vi "reset.vi"(8 "error in (no error)":errorcluster, 11 "DataCollectionDL110128Streaming in":refnum<class "DataCollectionDL110128Streaming.lvclass">) -> (0 "error out":errorcluster, 3 "DataCollectionDL110128Streaming out":refnum<class "DataCollectionDL110128Streaming.lvclass">)   [LabVIEW 2010, in "DataCollectionDL110128Streaming.lvclass"]
uses:
  DataCollectionDL110128Streaming.lvclass
  DataCollectionDL091104Scaffold/DataCollectionDL091104Scaffold/DataCollectionDL091104Scaffold.lvclass
  DataCollectionDL110128Streaming.lvclass/DataCollectionDL110128Streaming.ctl
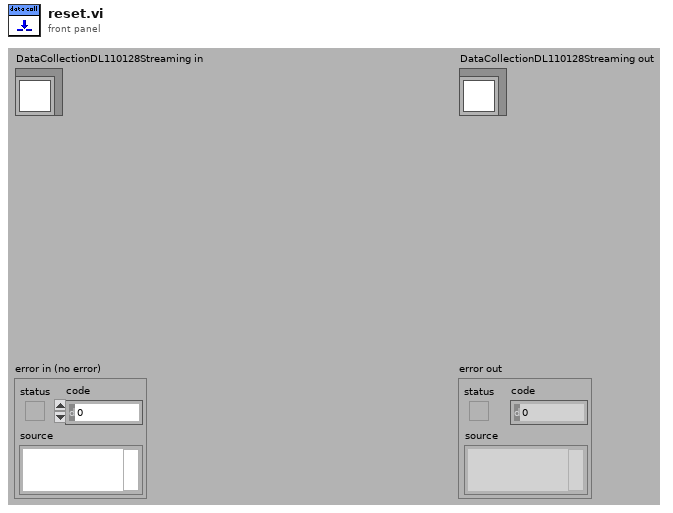
[diagram p1: front panel]
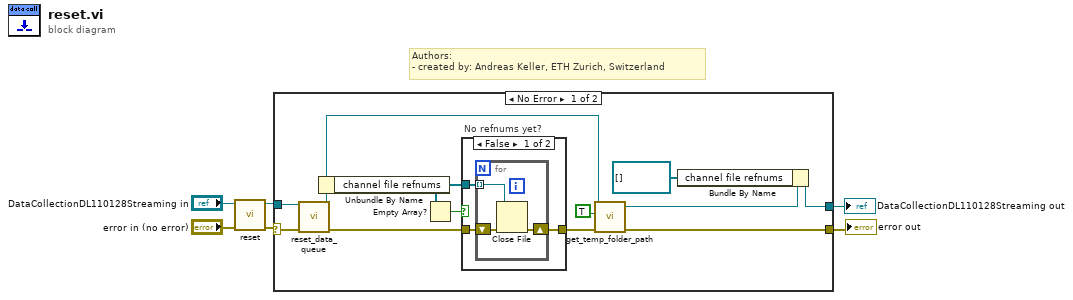
[diagram p0: block diagram]
diagram:
  # "Authors: \n- created by: Andreas Keller, ETH Zurich, Switzerland"
  n1 = call-parent "reset.vi"("error in (no error)"="error in (no error)", "DataCollectionDL091104Scaffold in"="DataCollectionDL110128Streaming in") -> ("error out"=w4:errorcluster, "DataCollectionDL091104Scaffold out"=w3:refnum<class "DataCollectionDL110128Streaming.lvclass">)  [unwired: 8 in]
  n2 = case shown="No Error" w4 {
    selector: w4 -> [w17 w27]
    tunnel: [w11 w27] -> w1
    tunnel: [w8 w26] -> w2
    tunnel: w3 -> [w18 w26]
    frame No Error {
      n3 = call-dynamic "reset_data_queue.vi"("error in (no error)"=w17, "GenericToplevelComponent in"=w18) -> ("error out"=w16:errorcluster, "GenericToplevelComponent out"=w10:refnum<class "DataCollectionDL110128Streaming.lvclass">)  [unwired: 8 in]
      n4 = Unbundle By Name(w10) -> ("channel file refnums"=w12:refnum<file>[])
      n5 = Empty Array?(array=w12) -> (empty?=w13:bool)
      n6 = case "No refnums yet?" shown="False" w13 {
        tunnel: w16 -> [w21 w25]
        tunnel: [w19 w25] -> w14
        tunnel: w12 -> [w20 _]
        frame False {
          n7 = for {
            tunnel: w20 -> [w23] mode=indexing
            shift-right: [w22] -> w19
            shift-left: w21 -> [w24]
            n8 = Close File(refnum=w23, error in=w24) -> (error out=w22:errorcluster)  [unwired: 1 out]
          }
        }
        frame True {
        }
      }
      n9 = call-dynamic "get_temp_folder_path.vi"("error in (no error)"=w14, "flush?"=TRUE, "GenericComponent in"=w10) -> ("error out"=w11:errorcluster, "GenericComponent out"=w9:refnum<class "DataCollectionDL110128Streaming.lvclass">)  [unwired: 6 in, 1 out]
      n10 = Bundle By Name(cluster=w9, "channel file refnums"=refnum<file>[] []) -> (w8:refnum<class "DataCollectionDL110128Streaming.lvclass">)
    }
    frame Error {
    }
  }
  "error out" <- w1
  "DataCollectionDL110128Streaming out" <- w2
